vi "Receive User Menu Selection Event.vi"(8 "error in (no error)":errorcluster, 10 "MenuSelectionMsg":refnum<class "MenuSelectionMsg.lvclass">, 11 "ActorAutoRegistrationView In":refnum<class "EventHandlingActor.lvclass">) -> (0 "error out":errorcluster, 3 "ActorAutoRegistrationView Out":refnum<class "EventHandlingActor.lvclass">)   [LabVIEW 2017, in "Integration Test Launcher.lvlib" / "TestViewables.lvlib" / "EventHandlingActor.lvclass"]
doc: "<License>\nCopyright © 2020 Tymphany, LLC | All rights reserved\nwww.Tymphany.com\nHuijun <Huijun.Guo@Tymphany.com>\n</License>"
uses:
  <vilib>/gpm_packages/@cs/example/Integration Test/ActorAutoRegistrationView/EventHandlingActor.lvclass
  <vilib>/gpm_packages/@cs/mva-viewable/Source/ActorEvents/IEventAggregator Messages/MenuSelectionMsg/MenuSelectionMsg.lvclass
  <vilib>/gpm_packages/@cs/mva-viewable/Source/ActorEvents/IEventAggregator Messages/MenuSelectionMsg/MenuSelectionMsg.lvclass/MenuSelectionMsg.ctl
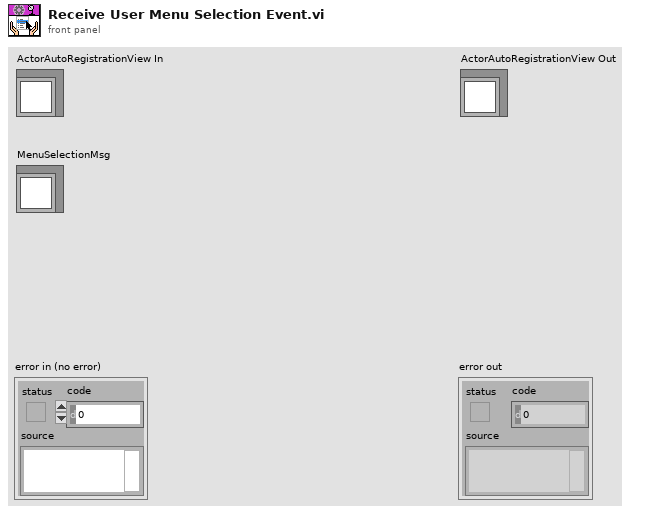
[diagram p1: front panel]
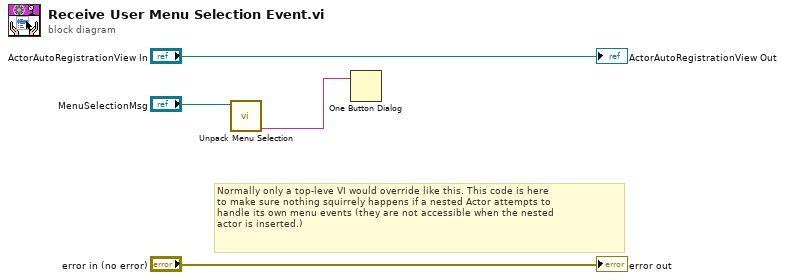
[diagram p0: block diagram]
diagram:
  # "Normally only a top-leve VI would override like this. This code is here\nto make sure nothing squirrely happens if a nested Actor attempts to\nhandle its own menu events (they are not accessible when the nested\nactor is inserted.)"
  n1 = call <vilib>:"Unpack Menu Selection.vi"("MenuSelectionMsg"="MenuSelectionMsg") -> ("Item Tag"=w2:string)  [unwired: 5 in, 5 out]
  n2 = One Button Dialog(message=w2) -> ()  [unwired: 1 in, 1 out]
  "error out" <- "error in (no error)"
  "ActorAutoRegistrationView Out" <- "ActorAutoRegistrationView In"
